vi "AVQ8347 Halfwidth Data.vi"(0 "VISA Session":refnum<visa-resource-name>, 5 "Error In":errorcluster) -> (12 "Return Data Bytes":u16, 13 "Fitting Error":dbl format="%.8e", 14 "Copy VISA Session":refnum<visa-resource-name>, 15 "Return All Data":string, 16 "CenterWaveLength":dbl format="%.8e", 17 "HalfWidth":dbl format="%.8e", 18 "Peak":i32, 19 "Error Out":errorcluster)   [LabVIEW 2021]
doc: "This function returns the halfwidth data value"
panel:
  out "String Work":string
  # "Halfwidth Data"
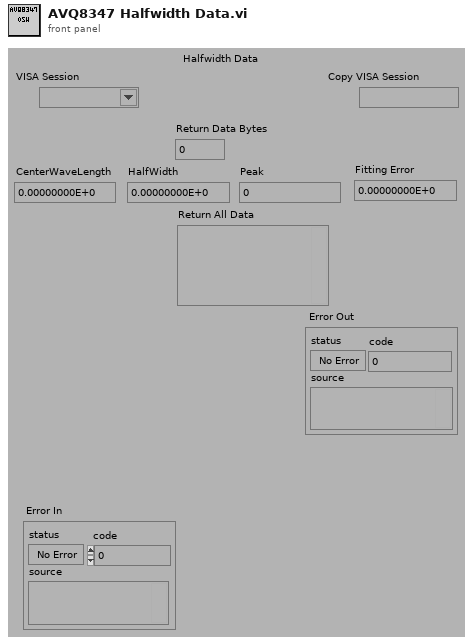
[diagram p1: front panel]
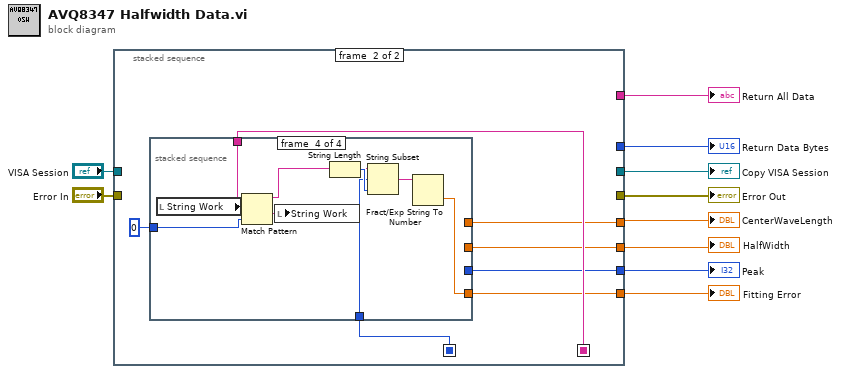
[diagram p0: block diagram]
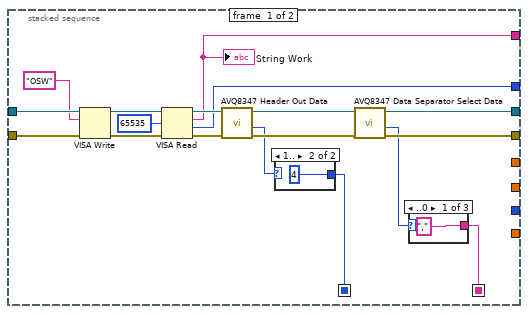
[diagram p2: hidden frame]
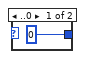
[diagram p3: hidden frame]
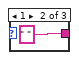
[diagram p4: hidden frame]
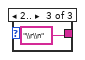
[diagram p5: hidden frame]
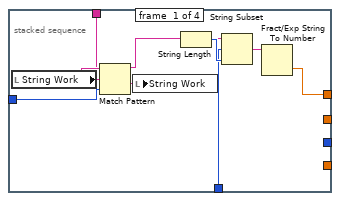
[diagram p6: hidden frame]
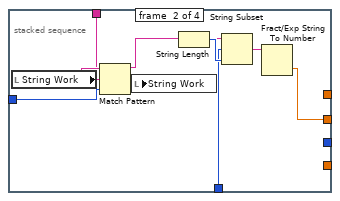
[diagram p7: hidden frame]
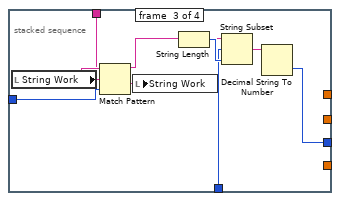
[diagram p8: hidden frame]
diagram:
  n1 = stacked-sequence {
    seq-local: [w27 _] -> [_ w39]
    seq-local: [w21 _] -> [_ w38]
    tunnel: "Error In" -> [w20 _]
    tunnel: "VISA Session" -> [w26 _]
    tunnel: [w14 _] -> w8
    tunnel: [w15 _] -> w7
    tunnel: [w17 _] -> w5
    tunnel: [w18 _] -> w6
    tunnel: [_ w37] -> w4
    tunnel: [_ w36] -> w3
    tunnel: [_ w35] -> w2
    tunnel: [_ w34] -> w1
    frame #0 {
      n2 = VISA Write(VISA resource name=w26, write buffer="OSW", error in (no error)=w20) -> (VISA resource name out=w22:refnum<visa-resource-name>, error out=w23:errorcluster)  [unwired: 1 out]
      n3 = VISA Read(VISA resource name=w22, byte count=65535, error in (no error)=w23) -> (VISA resource name out=w19:refnum<visa-resource-name>, read buffer=w17:string, return count=w18:u32, error out=w28:errorcluster)
      "String Work" <- w17
      n4 = call "AVQ8347 Header Out Data.vi"("Error In"=w28, "VISA Session"=w19) -> ("Error Out"=w16:errorcluster, "Header Data Out Control Value"=w12:u16, "Copy VISA Session"=w13:refnum<visa-resource-name>)  [unwired: 6 in, 1 out]
      n5 = case shown="1.." w12 {
        tunnel: [0 4] -> w27
        frame ..0 {
        }
        frame 1.. {
        }
      }
      n6 = call "AVQ8347 Data Separator Select Data.vi"("Error In"=w16, "VISA Session"=w13) -> ("Error Out"=w15:errorcluster, "Data Separrator Select Value"=w11:u16, "Copy VISA Session"=w14:refnum<visa-resource-name>)  [unwired: 6 in, 1 out]
      n7 = case shown="..0" w11 {
        tunnel: ["," " " "\\r\\n"] -> w21
        frame ..0 {
        }
        frame 1 {
        }
        frame 2.. {
        }
      }
    }
    frame #1 {
      n8 = stacked-sequence {
        tunnel: 0 -> [w48 w57 w66 w70]
        tunnel: w39 -> [w42 w52 w60 w68]
        tunnel: w38 -> [w41 w51 w59 w72]
        tunnel: [_ _ w61 _] -> w37
        tunnel: [w43 _ _ _] -> w36
        tunnel: [_ w50 _ _] -> w35
        tunnel: [_ _ _ w71] -> w34
        frame #0 {
          n9 = local read "String Work"() -> (w49:string)
          n10 = Match Pattern(string=w49, regular expression=w41, offset (0)=w48) -> (before substring=w45:string, after substring=w47:string)  [unwired: 2 out]
          n11 = local write "String Work"(w47) -> ()
          n12 = String Length(string=w45) -> (length=w46:i32)
          n13 = String Subset(string=w45, offset (0)=w42, length (rest)=w46) -> (substring=w44:string)
          n14 = Fract/Exp String To Number(string=w44) -> (number=w43:dbl)  [unwired: 3 in, 1 out]
        }
        frame #1 {
          n15 = local read "String Work"() -> (w58:string)
          n16 = Match Pattern(string=w58, regular expression=w51, offset (0)=w57) -> (before substring=w54:string, after substring=w56:string)  [unwired: 2 out]
          n17 = local write "String Work"(w56) -> ()
          n18 = String Length(string=w54) -> (length=w55:i32)
          n19 = String Subset(string=w54, offset (0)=w52, length (rest)=w55) -> (substring=w53:string)
          n20 = Fract/Exp String To Number(string=w53) -> (number=w50:dbl)  [unwired: 3 in, 1 out]
        }
        frame #2 {
          n21 = local read "String Work"() -> (w67:string)
          n22 = Match Pattern(string=w67, regular expression=w59, offset (0)=w66) -> (before substring=w63:string, after substring=w65:string)  [unwired: 2 out]
          n23 = local write "String Work"(w65) -> ()
          n24 = String Length(string=w63) -> (length=w64:i32)
          n25 = String Subset(string=w63, offset (0)=w60, length (rest)=w64) -> (substring=w62:string)
          n26 = Decimal String To Number(string=w62) -> (number=w61:i32)  [unwired: 2 in, 1 out]
        }
        frame #3 {
          n27 = local read "String Work"() -> (w69:string)
          n28 = Match Pattern(string=w69, regular expression=w72, offset (0)=w70) -> (before substring=w74:string, after substring=w76:string)  [unwired: 2 out]
          n29 = local write "String Work"(w76) -> ()
          n30 = String Length(string=w74) -> (length=w75:i32)
          n31 = String Subset(string=w74, offset (0)=w68, length (rest)=w75) -> (substring=w73:string)
          n32 = Fract/Exp String To Number(string=w73) -> (number=w71:dbl)  [unwired: 3 in, 1 out]
        }
      }
    }
  }
  "Return Data Bytes" <- w6
  "Return All Data" <- w5
  "Error Out" <- w7
  "Copy VISA Session" <- w8
  "CenterWaveLength" <- w3
  "HalfWidth" <- w2
  "Peak" <- w4
  "Fitting Error" <- w1
